vi "CRYReport Part LIB.vi"(7 "sAction":string, 8 "nData":i32, 9 "sData":string, 10 "cView":T2, 11 "cFrame":T1) -> (0 "nData_Out":i32, 1 "sData_Out":string, 2 "cView_Out":T2, 3 "cFrame_Out":T1)   [LabVIEW 2013]
uses:
  CRYReport Global.vi
  CRYWindow/DataView/VIEW/CRYView Global.vi
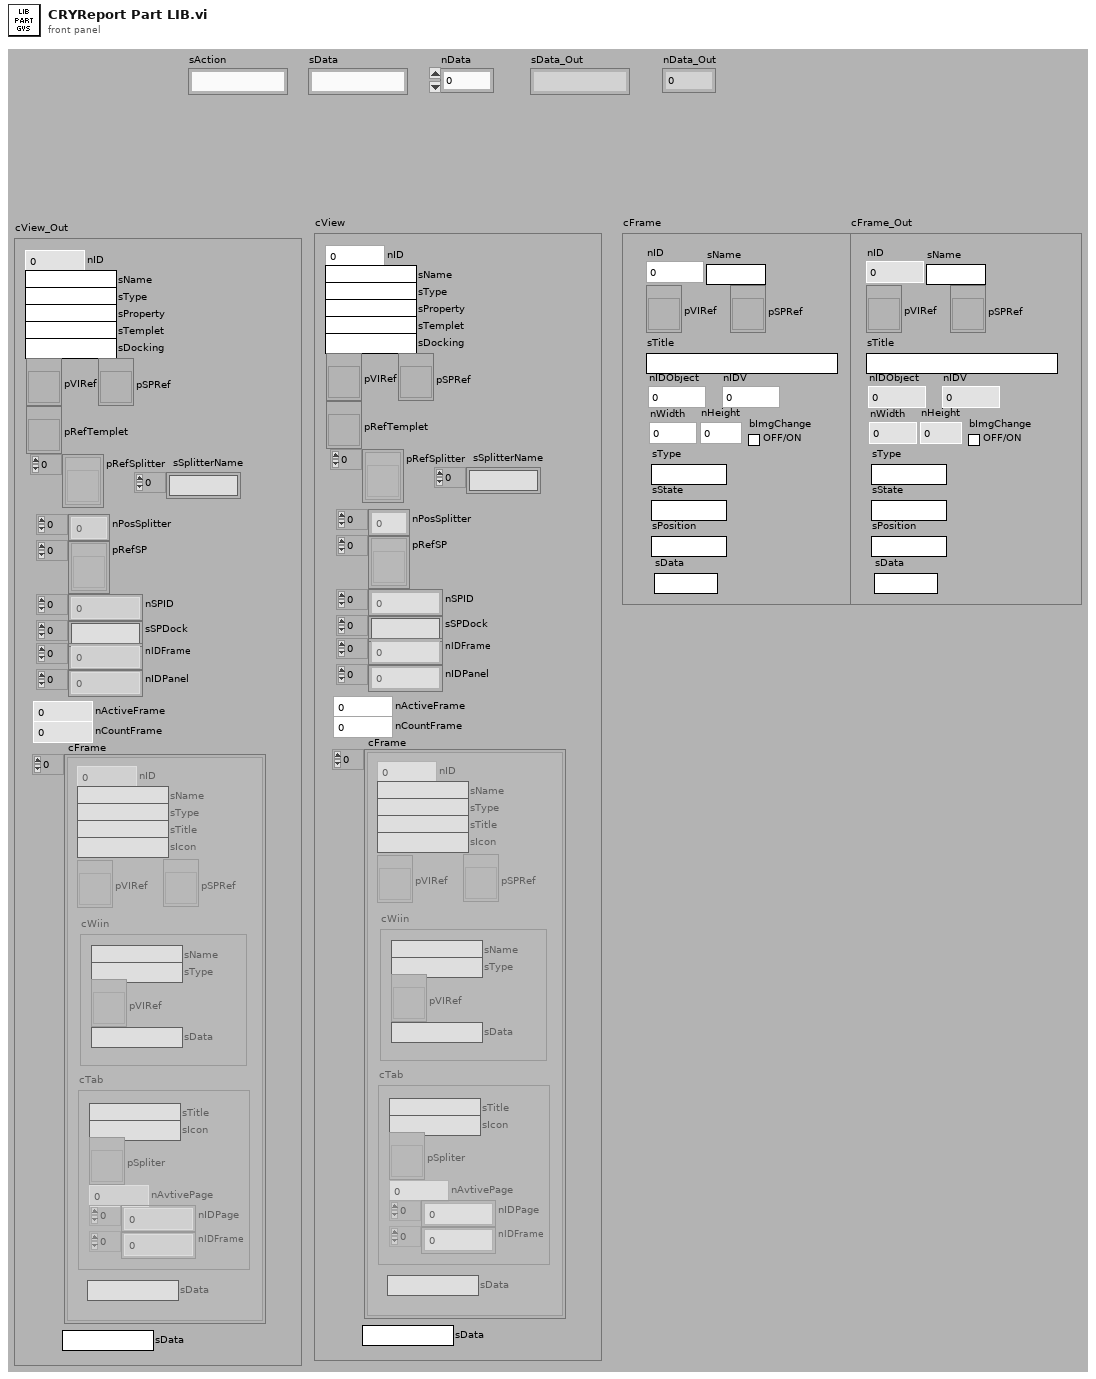
[diagram p1: front panel]
types:
  T1 = cluster{"nID":i16, "sName":string, "pVIRef":refnum<vi>, "pSPRef":refnum<vi>, "sTitle":string, "nIDObject":i16, "nIDV":i16, "nWidth":i16, "nHeight":i16, "bImgChange":bool, "sType":string, "sState":string, "sPosition":string, "sData":string}
  T2 = cluster{"nID":i32, "sName":string, "sType":string, "sProperty":string, "sTemplet":string, "sDocking":string, "pVIRef":refnum<vi>, "pSPRef":refnum<vi>, "pRefTemplet":refnum<vi>, "pRefSplitter":refnum<vi>[], "nPosSplitter":i32[], "pRefSP":refnum<vi>[], "nSPID":i32[], "sSPDock":string[], "nIDFrame":i32[], "nIDPanel":i32[], "nActiveFrame":i32, "nCountFrame":i32, "cFrame":cluster{"nID":i32, "sName":string, "sType":string, "sTitle":string, "sIcon":string, "pVIRef":refnum<vi>, "pSPRef":refnum<vi>, "cWiin":cluster{"sName":string, "sType":string, "pVIRef":refnum<vi>, "sData":string}, "cTab":cluster{"sTitle":string, "sIcon":string, "pSpliter":refnum<vi>, "nAvtivePage":i32, "nIDPage":i32[], "nIDFrame":i32[]}, "sData":string}[], "sData":string, "sSplitterName":string[]}
  T3 = enum32{"Invalid", "Standard", "Closed", "Hidden", "Minimized", "Maximized"}
  T4 = cluster{"sAction":string, "sType":string, "sQueueName":string, "sGraphName":string, "sData":string, "nData":i32, "pVIRef":refnum<vi>, "pSPRef":refnum<vi>}
  T5 = cluster{"nID":i32, "sName":string, "sType":string, "sProperty":string, "sTemplet":string, "sDocking":string, "pVIRef":refnum<vi>, "pSPRef":refnum<vi>, "pRefTemplet":refnum<vi>, "pRefSplitter":refnum<vi>[], "nPosSplitter":i32[], "pRefSP":refnum<vi>[], "nSPID":i32[], "sSPDock":string[], "nIDFrame":i32[], "nIDPanel":i32[], "nActiveFrame":i32, "nCountFrame":i32, "cFrame":cluster{"nID":i32, "sName":string, "sType":string, "sTitle":string, "sIcon":string, "pVIRef":refnum<vi>, "pSPRef":refnum<vi>, "cWin":cluster{"sName":string, "sType":string, "pVIRef":refnum<vi>, "sData":string}, "cTab":cluster{"sTitle":string, "sIcon":string, "pSpliter":refnum<vi>, "nAvtivePage":i32, "nIDPage":i32[], "nIDFrame":i32[]}, "sData":string}[], "sData":string, "sSplitterName":string[]}
  T6 = cluster{"sAction":string, "sData":string, "nData":i32, "pVIRef":refnum<vi>}
  T7 = cluster{"nCount":i16, "cFrameList":cluster{"nID":i16, "sName":string, "pVIRef":refnum<vi>, "pSPRef":refnum<vi>, "sTitle":string, "nIDObject":i16, "nIDV":i16, "nWidth":i16, "nHeight":i16, "bImgChange":bool, "sType":string, "sState":string, "sPosition":string, "sData":string}[], "sData":string}
  T8 = cluster{"nID":i16, "sName":string, "pVIRef":refnum<vi>, "pSPRef":refnum<vi>, "sTitle":string, "nIDObject":i16, "nIDV":i16, "nWidth":i16, "nHeight":i16, "bImgChange":bool, "sType":string, "sState":string, "sPosition":string, "sData":string}[]
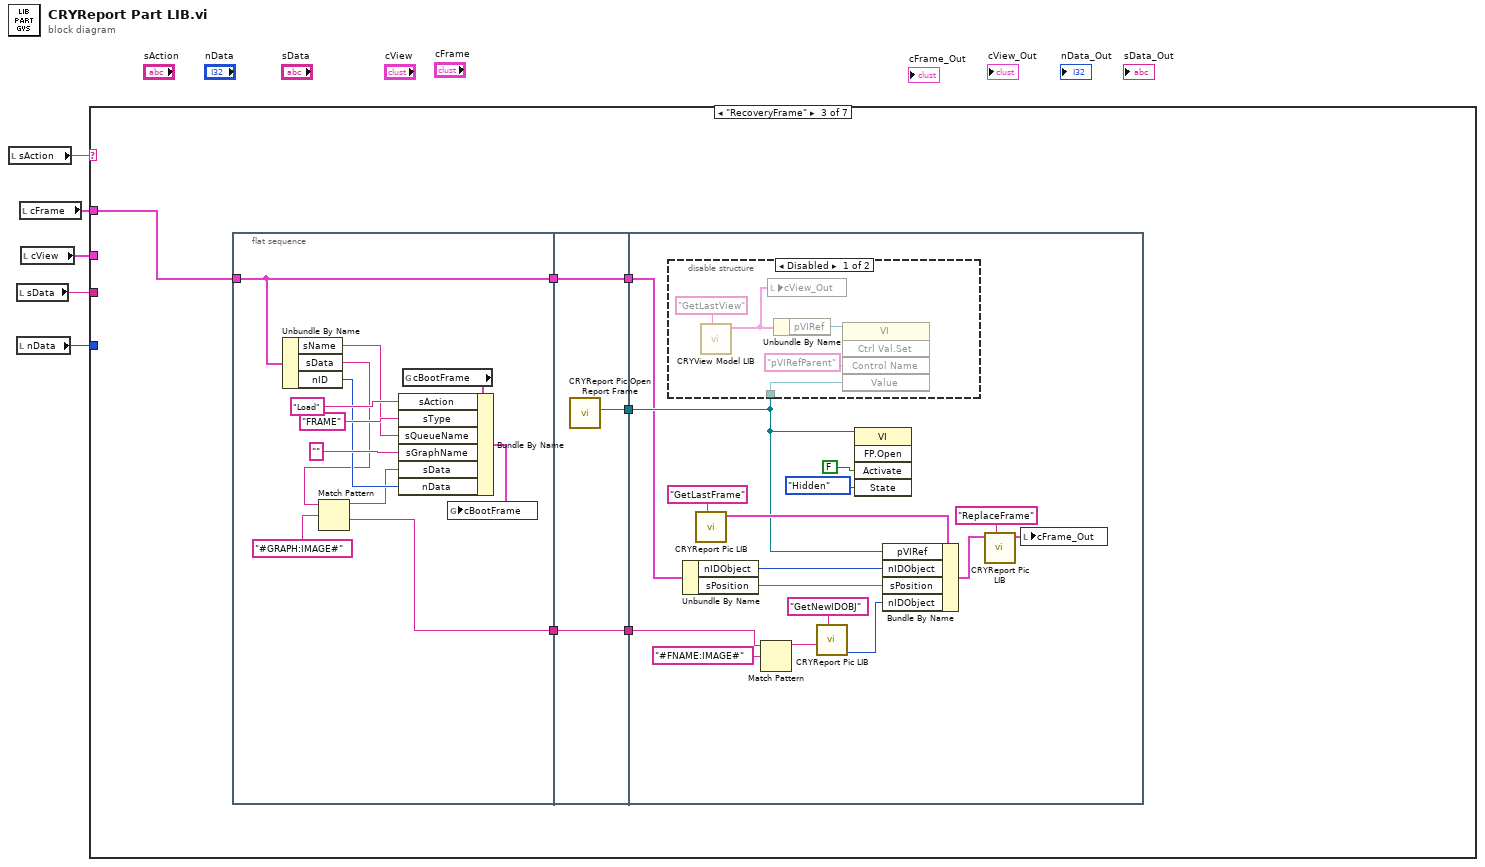
[diagram p0: block diagram]
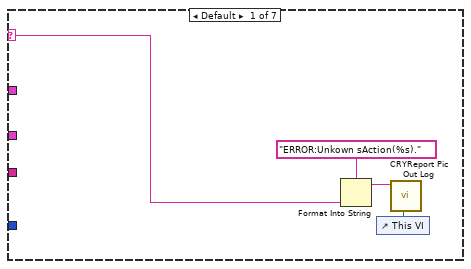
[diagram p2: hidden frame]
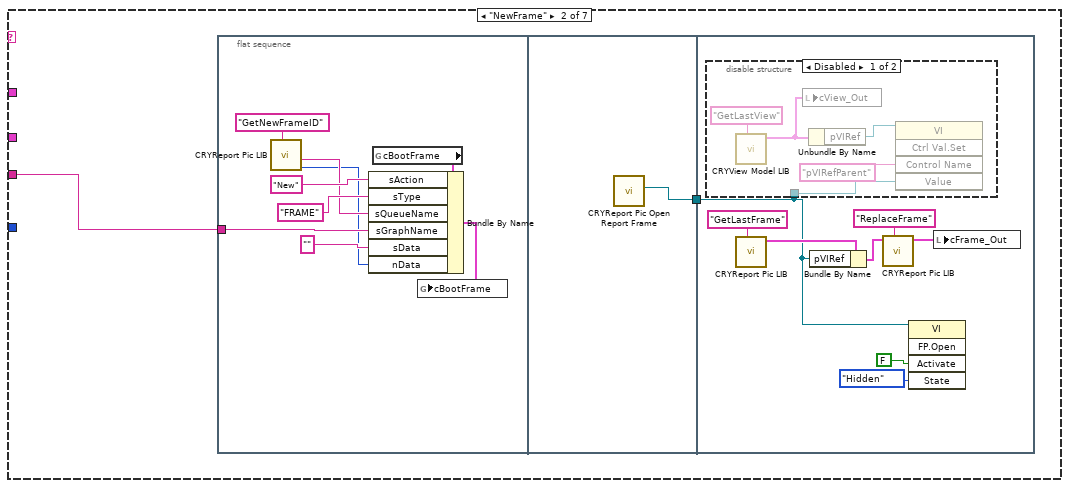
[diagram p3: hidden frame]
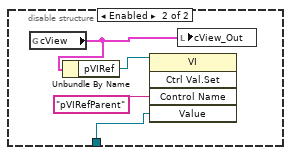
[diagram p4: hidden frame]
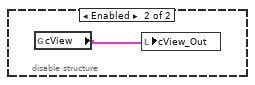
[diagram p5: hidden frame]
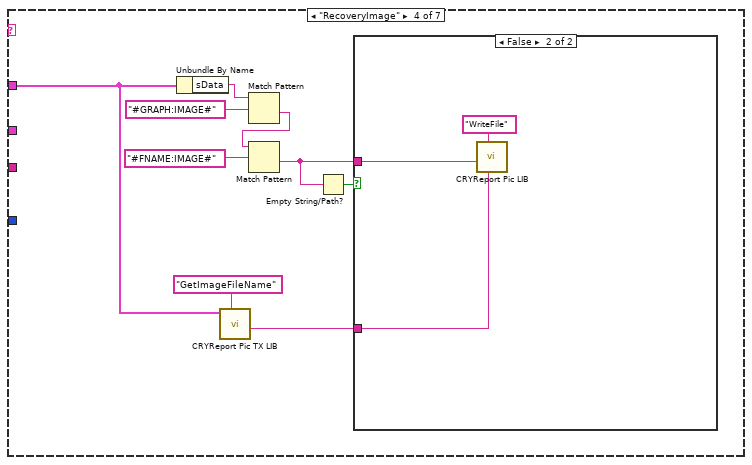
[diagram p6: hidden frame]
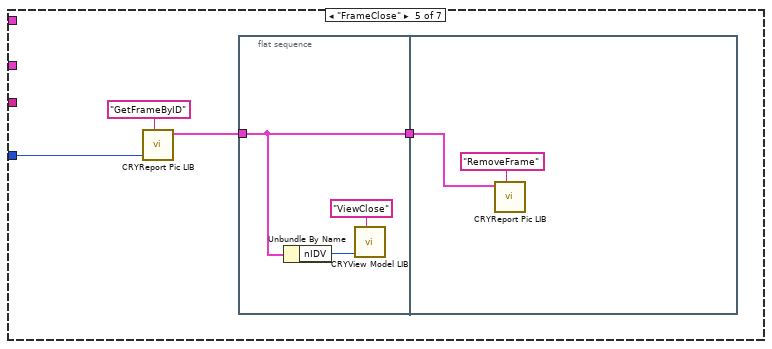
[diagram p8: hidden frame]
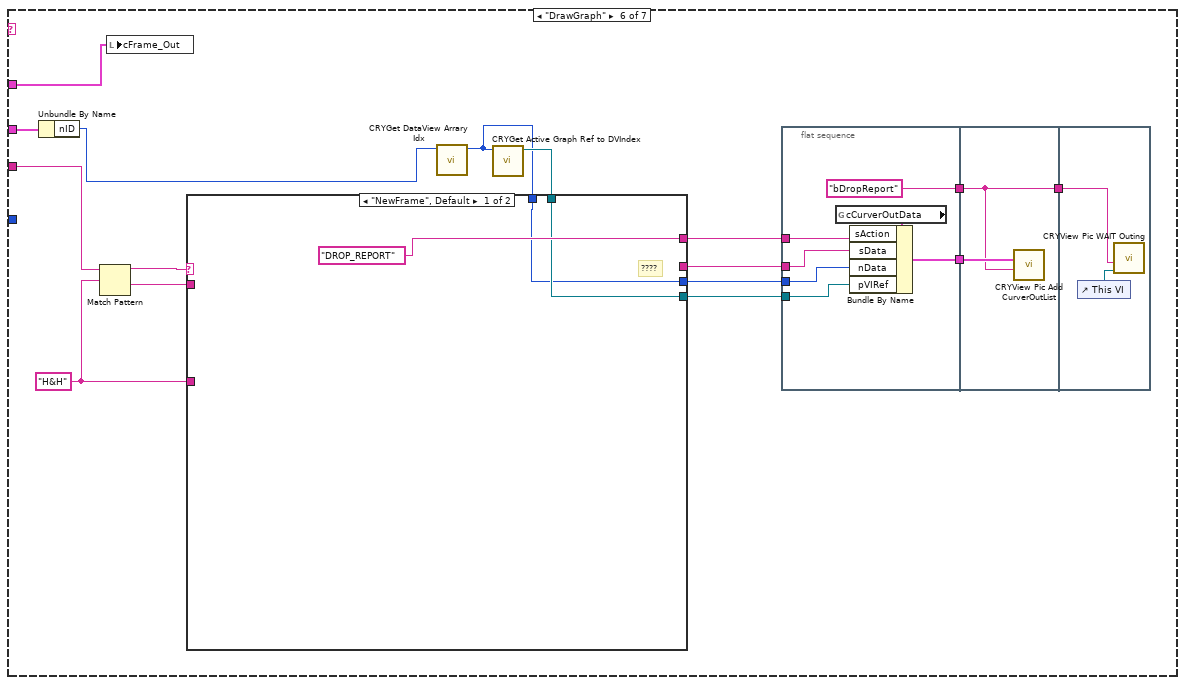
[diagram p9: hidden frame]
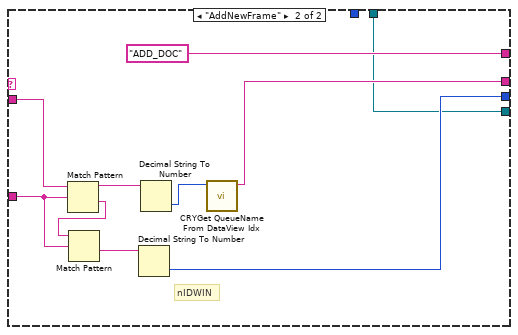
[diagram p10: hidden frame]
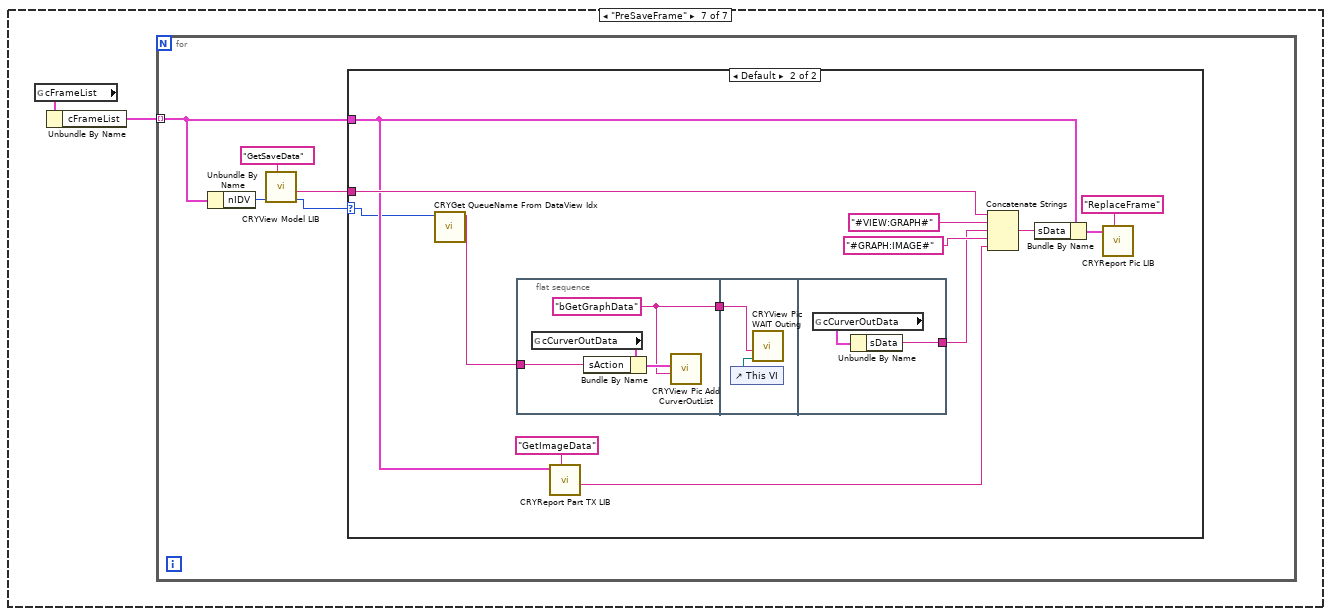
[diagram p11: hidden frame]
diagram:
  n1 = local read "sAction"() -> (w5:string)
  n2 = local read "sData"() -> (w4:string)
  n3 = local read "nData"() -> (w3:i32)
  n4 = local read "cFrame"() -> (w2:T1)
  n5 = local read "cView"() -> (w1:T2)
  n6 = case shown="\"RecoveryFrame\"" w5 {
    selector: w5 -> [w7 _ _ _ _ _ _]
    tunnel: w4 -> [_ w10 _ _ _ w114 _]
    tunnel: w3 -> [_ _ _ _ w96 _ _]
    tunnel: w2 -> [_ _ w43 w88 _ w118 _]
    tunnel: w1 -> [_ _ _ _ _ w104 _]
    frame Default {
      n7 = Format Into String(format string="ERROR:Unkown sAction(%s).", w7) -> (resulting string=w6:string)  [unwired: 2 in, 1 out]
      n8 = control-ref of="This VI"() -> (w9:refnum<vi>)
      n9 = call "CRYReport Pic Out Log.vi"("vi reference"=w9, "sData"=w6) -> ()  [unwired: 10 in]
    }
    frame "NewFrame" {
      n10 = flat-sequence {
        tunnel: w10 -> [w15]
        tunnel: [w21] -> w11
        tunnel: w11 -> [w22]
        frame #0 {
          n11 = call "CRYReport Pic LIB.vi"("sAction"="GetNewFrameID") -> ("nData_Out"=w12:i32, "sData_Out"=w13:string)  [unwired: 7 in, 2 out]
          n12 = global read "CRYReport Global.vi" "cBootFrame"() -> (w20:T4)
          n13 = Bundle By Name(cluster=w20, "sAction"="New", "sType"="FRAME" ("sQueueName"), "sQueueName"=w13, "sGraphName"=w15, "sData"="", "nData"=w12) -> (w16:T4)
          n14 = global write "CRYReport Global.vi" "cBootFrame"(w16) -> ()
        }
        frame #1 {
          n15 = call "CRYReport Pic Open Report Frame.vi"() -> ("pVIRef_Out"=w21:refnum<vi>)  [unwired: 11 in]
        }
        frame #2 {
          n16 = disable-structure shown="Disabled" {
            disable-tunnel: w22 -> [w30 w35]
            frame Disabled {
              n17 = call "CRYView Model LIB.vi"("sAction"="GetLastView") -> ("cView_Out"=w31:T2)  [unwired: 8 in, 2 out]
              n18 = local write "cView_Out"(w31) -> ()
              n19 = Unbundle By Name(w31) -> ("pVIRef"=w33:refnum<vi>)
              n20 = invoke class="VI" method="Ctrl Val.Set"(reference=w33, "Control Name"="pVIRefParent", "Value"=w30) -> ()  [unwired: 2 in, 5 out]
            }
            frame Enabled {
              n21 = global read "CRYView Global.vi" "cView"() -> (w36:T5)
              n22 = Unbundle By Name(w36) -> ("pVIRef"=w38:refnum<vi>)
              n23 = invoke class="VI" method="Ctrl Val.Set"(reference=w38, "Control Name"="pVIRefParent", "Value"=w35) -> ()  [unwired: 2 in, 5 out]
              n24 = local write "cView_Out"(w36) -> ()
            }
          }
          n25 = call "CRYReport Pic LIB.vi"("sAction"="GetLastFrame") -> ("cFrame_Out"=w28:T1)  [unwired: 7 in, 3 out]
          n26 = Bundle By Name(cluster=w28, "pVIRef"=w22) -> (w26:T1)
          n27 = call "CRYReport Pic LIB.vi"("sAction"="ReplaceFrame", "cFrame"=w26) -> ("cFrame_Out"=w25:T1)  [unwired: 6 in, 3 out]
          n28 = invoke class="VI" method="FP.Open"(reference=w22, "Activate"=FALSE ("Activate?"), "State"=T3."Hidden") -> ()  [unwired: 2 in, 5 out]
          n29 = local write "cFrame_Out"(w25) -> ()
        }
      }
    }
    frame "RecoveryFrame" {
      n30 = flat-sequence {
        tunnel: w43 -> [w49]
        tunnel: [w49] -> w41
        tunnel: [w45] -> w39
        tunnel: [w58] -> w44
        tunnel: [w59] -> w42
        tunnel: w41 -> [w59]
        tunnel: [w57] -> w40
        tunnel: w39 -> [w57]
        tunnel: w44 -> [w69]
        tunnel: w42 -> [w68]
        tunnel: w40 -> [w60]
        frame #0 {
          n31 = Unbundle By Name(w49) -> ("sName"=w51:string, "sData"=w46:string, "nID"=w50:i16)
          n32 = Match Pattern(string=w46, regular expression="#GRAPH:IMAGE#") -> (before substring=w47:string, after substring=w45:string)  [unwired: 1 in, 2 out]
          n33 = global read "CRYReport Global.vi" "cBootFrame"() -> (w56:T4)
          n34 = Bundle By Name(cluster=w56, "sAction"="Load", "sType"="FRAME" ("sQueueName"), "sQueueName"=w51, "sGraphName"="" ("sData"), "sData"=w47, "nData"=w50) -> (w53:T4)
          n35 = global write "CRYReport Global.vi" "cBootFrame"(w53) -> ()
        }
        frame #1 {
          n36 = call "CRYReport Pic Open Report Frame.vi"() -> ("pVIRef_Out"=w58:refnum<vi>)  [unwired: 11 in]
        }
        frame #2 {
          n37 = disable-structure shown="Disabled" {
            disable-tunnel: w69 -> [w76 _]
            frame Disabled {
              n38 = call "CRYView Model LIB.vi"("sAction"="GetLastView") -> ("cView_Out"=w77:T2)  [unwired: 8 in, 2 out]
              n39 = local write "cView_Out"(w77) -> ()
              n40 = Unbundle By Name(w77) -> ("pVIRef"=w79:refnum<vi>)
              n41 = invoke class="VI" method="Ctrl Val.Set"(reference=w79, "Control Name"="pVIRefParent", "Value"=w76) -> ()  [unwired: 2 in, 5 out]
            }
            frame Enabled {
              n42 = global read "CRYView Global.vi" "cView"() -> (w81:T5)
              n43 = local write "cView_Out"(w81) -> ()
            }
          }
          n44 = Unbundle By Name(w68) -> ("nIDObject"=w67:i16, "sPosition"=w66:string)
          n45 = call "CRYReport Pic LIB.vi"("sAction"="GetLastFrame") -> ("cFrame_Out"=w74:T1)  [unwired: 7 in, 3 out]
          n46 = Match Pattern(string=w60, regular expression="#FNAME:IMAGE#") -> (before substring=w61:string)  [unwired: 1 in, 3 out]
          n47 = call "CRYReport Pic LIB.vi"("sAction"="GetNewIDOBJ", "sData"=w61) -> ("nData_Out"=w63:i32)  [unwired: 6 in, 3 out]
          n48 = invoke class="VI" method="FP.Open"(reference=w69, "Activate"=FALSE ("Activate?"), "State"=T3."Hidden") -> ()  [unwired: 2 in, 5 out]
          n49 = Bundle By Name(cluster=w74, "pVIRef"=w69, "nIDObject"=w67, "sPosition"=w66, "nIDObject"=w63) -> (w65:T1)
          n50 = call "CRYReport Pic LIB.vi"("sAction"="ReplaceFrame", "cFrame"=w65) -> ("cFrame_Out"=w72:T1)  [unwired: 6 in, 3 out]
          n51 = local write "cFrame_Out"(w72) -> ()
        }
      }
    }
    frame "RecoveryImage" {
      n52 = Unbundle By Name(w88) -> ("sData"=w90:string)
      n53 = call "CRYReport Pic TX LIB.vi"("sAction"="GetImageFileName", "cFrame"=w88) -> ("sData_Out"=w86:string)  [unwired: 7 in, 2 out]
      n54 = Match Pattern(string=w90, regular expression="#GRAPH:IMAGE#") -> (after substring=w83:string)  [unwired: 1 in, 3 out]
      n55 = Match Pattern(string=w83, regular expression="#FNAME:IMAGE#") -> (after substring=w82:string)  [unwired: 1 in, 3 out]
      n56 = Empty String/Path?(string/path=w82) -> (empty?=w87:bool)
      n57 = case shown="False" w87 {
        tunnel: w82 -> [_ w91]
        tunnel: w86 -> [_ w92]
        frame True {
        }
        frame False {
          n58 = call "CRYReport Pic LIB.vi"("sOption"=w92, "sAction"="WriteFile", "sData"=w91) -> ()  [unwired: 5 in, 4 out]
        }
      }
    }
    frame "FrameClose" {
      n59 = call "CRYReport Pic LIB.vi"("sAction"="GetFrameByID", "nData"=w96) -> ("cFrame_Out"=w94:T1)  [unwired: 6 in, 3 out]
      n60 = flat-sequence {
        tunnel: w94 -> [w98]
        tunnel: [w98] -> w95
        tunnel: w95 -> [w101]
        frame #0 {
          n61 = Unbundle By Name(w98) -> ("nIDV"=w99:i16)
          n62 = call "CRYView Model LIB.vi"("sAction"="ViewClose", "nData"=w99) -> ()  [unwired: 7 in, 3 out]
        }
        frame #1 {
          n63 = call "CRYReport Pic LIB.vi"("sAction"="RemoveFrame", "cFrame"=w101) -> ()  [unwired: 6 in, 4 out]
        }
      }
    }
    frame "DrawGraph" {
      w107 = "H&H"
      n64 = Unbundle By Name(w104) -> ("nID"=w103:i32)
      n65 = Match Pattern(string=w114, regular expression=w107) -> (before substring=w113:string, after substring=w112:string)  [unwired: 1 in, 2 out]
      n66 = local write "cFrame_Out"(w118) -> ()
      n67 = call "CRYGet DataView Arrary Idx.vi"("DataView Idx In"=w103) -> ("DataView Arrary Idx out"=w105:i32)  [unwired: 10 in]
      n68 = call "CRYGet Active Graph Ref to DVIndex.vi"("DV Array index"=w105) -> ("Inserted Graph VIRef out"=w106:refnum<vi>)  [unwired: 5 in, 5 out]
      n69 = case shown="\"NewFrame\", Default" w113 {
        tunnel: ["DROP_REPORT" ("sAction") "ADD_DOC" ("sAction")] -> w111
        tunnel: w112 -> [_ w130]
        tunnel: [_ w128] -> w110
        tunnel: [w119 w127] -> w109
        tunnel: [w120 w126] -> w108
        tunnel: w107 -> [_ w129]
        tunnel: w106 -> [w120 w126]
        tunnel: w105 -> [w119 _]
        frame "NewFrame", Default {
          # "????"
        }
        frame "AddNewFrame" {
          # "nIDWIN"
          n70 = Match Pattern(string=w130, regular expression=w129) -> (before substring=w123:string, after substring=w125:string)  [unwired: 1 in, 2 out]
          n71 = Match Pattern(string=w125, regular expression=w129) -> (after substring=w124:string)  [unwired: 1 in, 3 out]
          n72 = Decimal String To Number(string=w124) -> (number=w127:i32)  [unwired: 2 in, 1 out]
          n73 = Decimal String To Number(string=w123) -> (number=w122:i32)  [unwired: 2 in, 1 out]
          n74 = call "CRYGet QueueName From DataView Idx.vi"("DataView Idx"=w122) -> ("DataView sQueueName"=w128:string)  [unwired: 10 in]
        }
      }
      n75 = flat-sequence {
        tunnel: w111 -> [w137]
        tunnel: w108 -> [w136]
        tunnel: ["bDropReport" ("Label Name")] -> w117
        tunnel: w109 -> [w134]
        tunnel: w110 -> [w133]
        tunnel: [w132] -> w115
        tunnel: w117 -> [w139]
        tunnel: [w139] -> w116
        tunnel: w115 -> [w140]
        tunnel: w116 -> [w141]
        frame #0 {
          n76 = global read "CRYView Global.vi" "cCurverOutData"() -> (w138:T6)
          n77 = Bundle By Name(cluster=w138, "sAction"=w137, "sData"=w133, "nData"=w134, "pVIRef"=w136) -> (w132:T6)
        }
        frame #1 {
          n78 = call "CRYView Pic Add CurverOutList.vi"("sName"=w139, "cCurverOutData"=w140) -> ()  [unwired: 10 in]
        }
        frame #2 {
          n79 = control-ref of="This VI"() -> (w142:refnum<vi>)
          n80 = call "CRYView Pic WAIT Outing.vi"("pVIRef"=w142, "sData"=w141) -> ()  [unwired: 9 in, 1 out]
        }
      }
    }
    frame "PreSaveFrame" {
      n81 = global read "CRYReport Global.vi" "cFrameList"() -> (w144:T7)
      n82 = Unbundle By Name(w144) -> ("cFrameList"=w143:T8)
      n83 = for {
        tunnel: w143 -> [w146] mode=indexing
        n84 = Unbundle By Name(w146) -> ("nIDV"=w148:i16)
        n85 = call "CRYView Model LIB.vi"("sAction"="GetSaveData", "nData"=w148) -> ("nData_Out"=w145:i32, "sData_Out"=w147:string)  [unwired: 7 in, 1 out]
        n86 = case shown="Default" w145 {
          selector: w145 -> [_ w151]
          tunnel: w147 -> [_ w161]
          tunnel: w146 -> [_ w154]
          frame -1 {
          }
          frame Default {
            n87 = call "CRYGet QueueName From DataView Idx.vi"("DataView Idx"=w151) -> ("DataView sQueueName"=w150:string)  [unwired: 10 in]
            n88 = flat-sequence {
              tunnel: [w163] -> w152
              tunnel: w150 -> [w165]
              tunnel: w152 -> [w167]
              tunnel: [w169] -> w153
              frame #0 {
                w163 = "bGetGraphData" ("sData")
                n89 = global read "CRYView Global.vi" "cCurverOutData"() -> (w166:T6)
                n90 = Bundle By Name(cluster=w166, "sAction"=w165) -> (w164:T6)
                n91 = call "CRYView Pic Add CurverOutList.vi"("sName"=w163, "cCurverOutData"=w164) -> ()  [unwired: 10 in]
              }
              frame #1 {
                n92 = control-ref of="This VI"() -> (w168:refnum<vi>)
                n93 = call "CRYView Pic WAIT Outing.vi"("pVIRef"=w168, "sData"=w167) -> ()  [unwired: 9 in, 1 out]
              }
              frame #2 {
                n94 = global read "CRYView Global.vi" "cCurverOutData"() -> (w170:T6)
                n95 = Unbundle By Name(w170) -> ("sData"=w169:string)
              }
            }
            n96 = call "CRYReport Part TX LIB.vi"("sAction"="GetImageData", "cFrame"=w154) -> ("sData_Out"=w155:string)  [unwired: 7 in, 2 out]
            n97 = Concatenate Strings(w161, "#VIEW:GRAPH#" ("regular expression"), w153, "#GRAPH:IMAGE#" ("regular expression"), w155) -> (w160:string)
            n98 = Bundle By Name(cluster=w154, "sData"=w160) -> (w159:T1)
            n99 = call "CRYReport Pic LIB.vi"("sAction"="ReplaceFrame", "cFrame"=w159) -> ()  [unwired: 6 in, 4 out]
          }
        }
      }
    }
  }
